vi "Post_Trend Data.vi"(7 "LabVIEW Web Service Request":refnum<class "Web Request.lvclass">) -> ()   [LabVIEW 2016]
uses:
  <vilib>/wsapi/Web Request.lvclass
  Store Data/Data Library.lvlib
panel:
  out "value":T1
  # "Use the Web Service Request input terminal to call the VIs on the Web Services palette. Do not remove it from the connector pane unless you don't need access to the palette."
  # "Each additional control wired to the connector pane will be available as an input in the URL. To include an indicator in terminal-mode output (the default setting), it must also be wired to the connector pane."
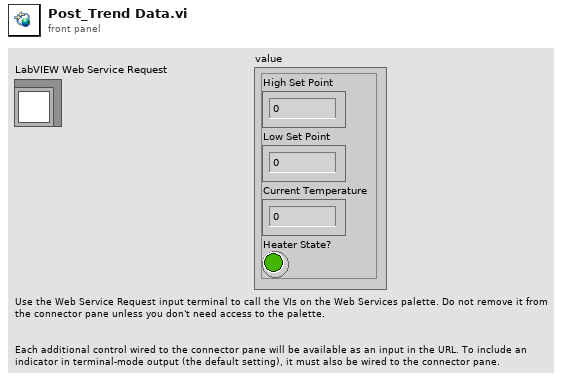
[diagram p1: front panel]
types:
  T1 = cluster{"High Set Point":dbl, "Low Set Point":dbl, "Current Temperature":dbl, "Heater State?":bool}
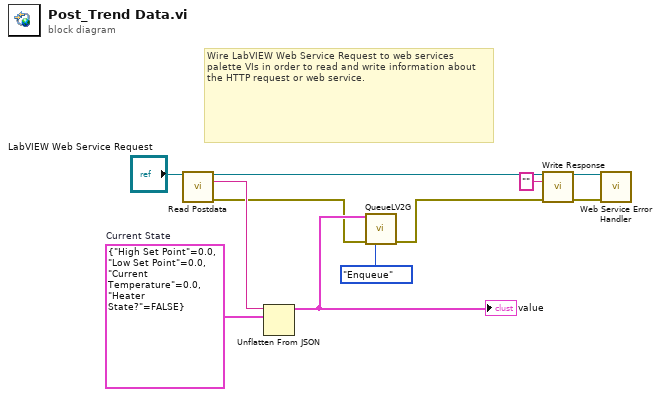
[diagram p0: block diagram]
diagram:
  w6 = T1 {"High Set Point"=0.0, "Low Set Point"=0.0, "Current Temperature"=0.0, "Heater State?"=FALSE}  # Current State
  # "Wire LabVIEW Web Service Request to web services palette VIs in order to read and write information about the HTTP request or web service."
  n1 = call <vilib>:"Read Postdata.vi"("LabVIEW Web Service Request"="LabVIEW Web Service Request") -> ("LabVIEW Web Service Request out"=w8:refnum<class "Web Request.lvclass">, "postdata"=w7:string, "error out"=w2:errorcluster)  [unwired: 12 in]
  n2 = Unflatten From JSON(JSON string=w7, type and defaults=w6) -> (value=w3:T1)  [unwired: 5 in, 1 out]
  "value" <- w3
  n3 = call "QueueLV2G.vi"("r"=w3, "error in (no error)"=w2, "Selector"=enum16{"Create", "Enqueue", "Status", "Destroy"}."Enqueue") -> ("error out"=w1:errorcluster)  [unwired: 11 in, 1 out]
  n4 = call <vilib>:"Write Response.vi"("LabVIEW Web Service Request"=w8, "response string"="", "error in (no error)"=w1) -> ("LabVIEW Web Service Request out"=w11:refnum<class "Web Request.lvclass">, "error out"=w10:errorcluster)  [unwired: 11 in]
  n5 = call "Web Service Error Handler.vi"("LabVIEW Web Service Request"=w11, "error in (no error)"=w10) -> ()  [unwired: 12 in, 2 out]
